vi "Get Data Type Information.vi"(8 "error in (no error)":errorcluster, 10 "Name":string, 11 "TwinCAT ADS in":refnum<class "TwinCAT ADS.lvclass">) -> (0 "error out":errorcluster, 1 "Data Type Info":refnum<k24>, 3 "TwinCAT ADS out":refnum<class "TwinCAT ADS.lvclass">)   [LabVIEW 2018, in "TwinCAT ADS.lvclass"]
uses:
  TwinCAT ADS.lvclass
  TwinCAT.Ads
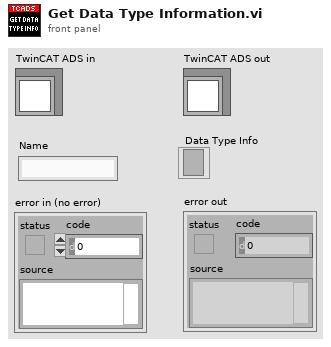
[diagram p1: front panel]
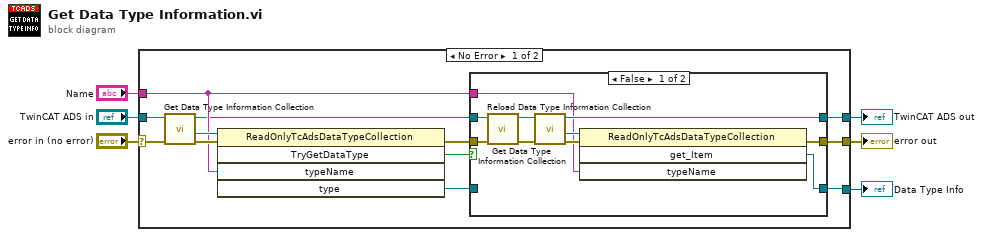
[diagram p0: block diagram]
diagram:
  n1 = case shown="No Error" "error in (no error)" {
    selector: "error in (no error)" -> [w12 w33]
    tunnel: [w15 w33] -> w5
    tunnel: [w14 w32] -> w3
    tunnel: "TwinCAT ADS in" -> [w13 w32]
    tunnel: "Name" -> [w9 _]
    tunnel: [w7 _] -> w1
    frame No Error {
      n2 = call-dynamic "Get Data Type Information Collection.vi"("error in (no error)"=w12, "TwinCAT ADS in"=w13) -> ("error out"=w10:errorcluster, "Data Type Info Collection"=w11:refnum<k24>, "TwinCAT ADS out"=w8:refnum<class "TwinCAT ADS.lvclass">)  [unwired: 7 in]
      n3 = invoke class="ReadOnlyTcAdsDataTypeCollection" method="TryGetDataType"(reference=w11, error in=w10, "typeName"=w9) -> (error out=w16:errorcluster, "TryGetDataType"=w18:bool, "type"=w17:refnum<k24>)  [unwired: 2 in, 2 out]
      n4 = case shown="False" w18 {
        tunnel: w17 -> [_ w31]
        tunnel: [w25 w31] -> w7
        tunnel: w16 -> [w28 w30]
        tunnel: w8 -> [w27 w29]
        tunnel: [w20 w29] -> w14
        tunnel: w9 -> [w19 _]
        tunnel: [w26 w30] -> w15
        frame False {
          n5 = call-dynamic "Reload Data Type Information Collection.vi"("error in (no error)"=w28, "TwinCAT ADS in"=w27) -> ("error out"=w24:errorcluster, "TwinCAT ADS out"=w23:refnum<class "TwinCAT ADS.lvclass">)  [unwired: 8 in]
          n6 = call-dynamic "Get Data Type Information Collection.vi"("error in (no error)"=w24, "TwinCAT ADS in"=w23) -> ("error out"=w22:errorcluster, "Data Type Info Collection"=w21:refnum<k24>, "TwinCAT ADS out"=w20:refnum<class "TwinCAT ADS.lvclass">)  [unwired: 7 in]
          n7 = invoke class="ReadOnlyTcAdsDataTypeCollection" method="get_Item"(reference=w21, error in=w22, "typeName"=w19) -> (error out=w26:errorcluster, "get_Item"=w25:refnum<k24>)  [unwired: 1 in, 2 out]
        }
        frame True {
        }
      }
    }
    frame Error {
    }
  }
  "error out" <- w5
  "TwinCAT ADS out" <- w3
  "Data Type Info" <- w1
